vi "Set GPU.vi"(8 "error in (no error)":errorcluster, 9 "Device ID":i32, 10 "Backend":T1 items=["Default Backend"=0, "CPU Backend"=1, "CUDA Backend"=2, "OPENCL Backend"=4, "Intel OneAPI"=8], 11 "GPU FFT Calculator in":refnum<class "GPU FFT Calculator.lvclass">) -> (0 "error out":errorcluster, 3 "GPU FFT Calculator out":refnum<class "GPU FFT Calculator.lvclass">)   [LabVIEW 2020, in "GPU FFT Calculator.lvlib" / "GPU FFT Calculator.lvclass"]
uses:
  GPU FFT Calculator.lvclass
  <vilib>/Natan Biesmans/G2CPU GPU and CPU HPC Toolkit/ArrayFire Driver/TypeDefs/backend.ctl
  QMH Message.ctl
  GPU Device Message.ctl
  GPU FFT Calculator.lvclass/GPU FFT Calculator.ctl
  <vilib>/Natan Biesmans/G2CPU GPU and CPU HPC Toolkit/ArrayFire Driver/AF.lvlib
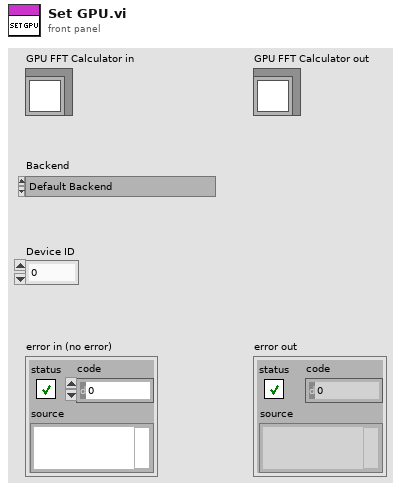
[diagram p1: front panel]
types:
  T1 = typedef "AF.lvlib/backend.ctl" = u32
  T2 = typedef "GPU FFT Calculator.lvlib/GPU FFT Calculator.lvclass/GPU Device Message.ctl" = cluster{"Backend":T1, "Device ID":i32}
  T3 = typedef "GPU FFT Calculator.lvlib/GPU FFT Calculator.lvclass/QMH Message.ctl" = cluster{"Command":string, "Data":variant}
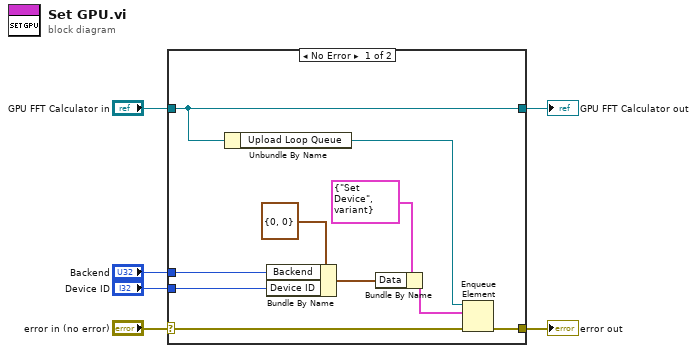
[diagram p0: block diagram]
diagram:
  n1 = case shown="No Error" "error in (no error)" {
    selector: "error in (no error)" -> [w14 w18]
    tunnel: [w13 w18] -> w5
    tunnel: [w16 w17] -> w3
    tunnel: "GPU FFT Calculator in" -> [w16 w17]
    tunnel: "Backend" -> [w8 _]
    tunnel: "Device ID" -> [w7 _]
    frame No Error {
      n2 = Unbundle By Name(w16) -> ("Upload Loop Queue"=w15:refnum<queue>)
      n3 = Bundle By Name(cluster=T2 {"Backend"=0, "Device ID"=0} ("Cluster"), "Backend"=w8, "Device ID"=w7) -> (w9:T2)
      n4 = Bundle By Name(cluster=T3 {"Command"="Set Device", "Data"=variant} ("element"), "Data"=w9) -> (w11:T3)
      n5 = Enqueue Element(queue=w15, element=w11, error in (no error)=w14) -> (error out=w13:errorcluster)  [unwired: 1 in, 2 out]
    }
    frame Error {
    }
  }
  "error out" <- w5
  "GPU FFT Calculator out" <- w3
